vi "GenerateTriggeredStimulus.vi"(8 "error in (no error)":errorcluster, 11 "Stimulus in":refnum<class "FullWormRailsTwoColors.lvclass">) -> (0 "error out":errorcluster, 2 "TriggeredStimulus":sgl[][](array[numeric]), 3 "Stimulus out":refnum<class "FullWormRailsTwoColors.lvclass">)   [LabVIEW 2019, in "FullWormRailsTwoColors.lvclass"]
uses:
  FullWormRailsTwoColors.lvclass
  FullWormRailsTwoColors.lvclass/FullWormRailsTwoColors.ctl
  <vilib>/numeric/Random Number (Range) U64.vi
  <vilib>/numeric/sub_Random U32.vi
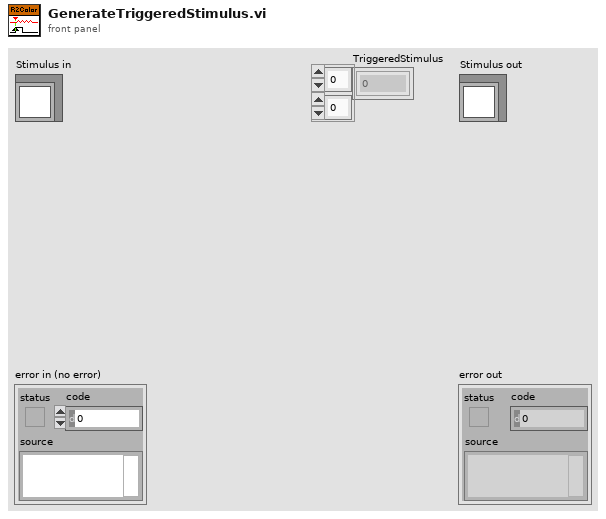
[diagram p1: front panel]
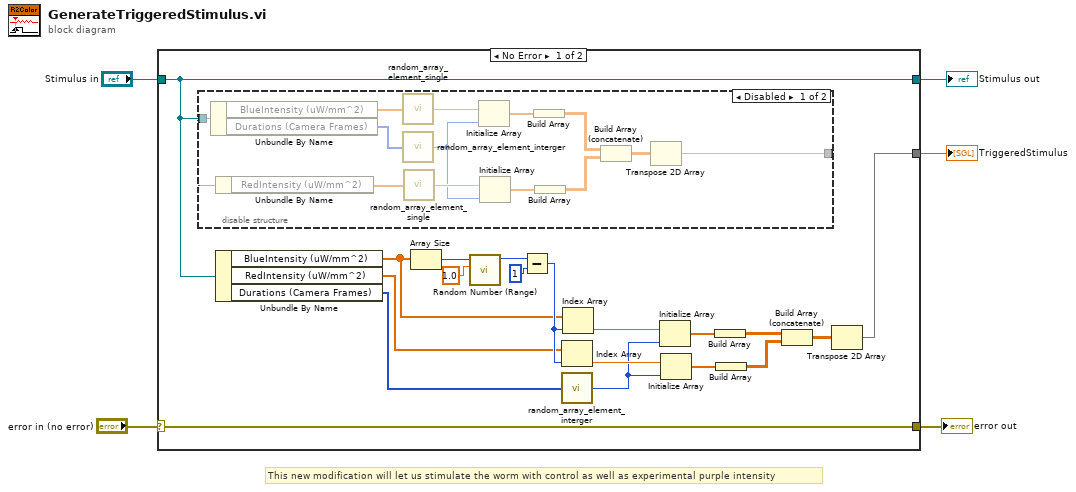
[diagram p0: block diagram]
diagram:
  # "This new modification will let us stimulate the worm with control as well as experimental purple intensity"
  n1 = case shown="No Error" "error in (no error)" {
    selector: "error in (no error)" -> [w24 w39]
    tunnel: [w24 w39] -> w1
    tunnel: [w7 w38] -> w4
    tunnel: "Stimulus in" -> [w7 w38]
    tunnel: [w6 _] -> w2
    frame No Error {
      n2 = disable-structure shown="Disabled" {
        disable-tunnel: [w30 _] -> _
        disable-tunnel: w7 -> [w25 _]
        frame Disabled {
          n3 = Unbundle By Name(w25) -> ("BlueIntensity (uW/mm^2)"=w37:sgl[], "Durations (Camera Frames)"=w27:i32[])
          n4 = Unbundle By Name(w25) -> ("RedIntensity (uW/mm^2)"=w33:sgl[])
          n5 = call "random_array_element_single.vi"("Array of numbers"=w37) -> ("Randomly selected number"=w36:sgl)
          n6 = call "random_array_element_interger.vi"("Array of numbers"=w27) -> ("Randomly selected number"=w26:i32)
          n7 = call "random_array_element_single.vi"("Array of numbers"=w33) -> ("Randomly selected number"=w32:sgl)
          n8 = Initialize Array(w36, w26) -> (w35:sgl[])
          n9 = Initialize Array(w32, w26) -> (w34:sgl[])
          n10 = Build Array(w35) -> (w29:sgl[][])
          n11 = Build Array(w34) -> (w28:sgl[][])
          n12 = Build Array (concatenate)(w29, w28) -> (w31:sgl[][])
          n13 = Transpose 2D Array(2D array=w31) -> (transposed array=w30:sgl[][])
        }
        frame Enabled {
        }
      }
      n14 = Unbundle By Name(w7) -> ("BlueIntensity (uW/mm^2)"=w10:sgl[], "RedIntensity (uW/mm^2)"=w9:sgl[], "Durations (Camera Frames)"=w8:i32[])
      n15 = Array Size(array=w10) -> (size(s)=w23:i32)
      n16 = call-poly <vilib>:"Random Number (Range).vi"("lower bound (0)"=1.0, "upper bound (100)"=w23) -> ("number"=w21:u64)  [unwired: 9 in]
      n17 = Subtract(x=w21, y=u64 1) -> (x-y=w11:u64)
      n18 = Index Array(array=w9, index=w11) -> (element=w13:sgl)
      n19 = call "random_array_element_interger.vi"("Array of numbers"=w8) -> ("Randomly selected number"=w12:i32)
      n20 = Index Array(array=w10, index=w11) -> (element=w14:sgl)
      n21 = Initialize Array(w14, w12) -> (w19:sgl[])
      n22 = Initialize Array(w13, w12) -> (w18:sgl[])
      n23 = Build Array(w19) -> (w16:sgl[][])
      n24 = Build Array(w18) -> (w15:sgl[][])
      n25 = Build Array (concatenate)(w16, w15) -> (w17:sgl[][])
      n26 = Transpose 2D Array(2D array=w17) -> (transposed array=w6:sgl[][])
    }
    frame Error {
    }
  }
  "error out" <- w1
  "Stimulus out" <- w4
  "TriggeredStimulus" <- w2
